vi "one.vi"() -> ()   [LabVIEW 2021]
uses:
  <vilib>/express/express analysis/Spectral/Block/exnSpectralBlock spectral measurements RMS poly.vi
  <vilib>/express/express analysis/Spectral/Block/exnSpectralBlock spectral measurements RMS DDT.vi
  <vilib>/express/express analysis/Spectral/XNode/ExpressSpectralMeasurementsBlockNode.xnode
panel:
  out "Graph in Time":dynamicdata(graph)
  out "Graph in Frequency":dynamicdata(graph)
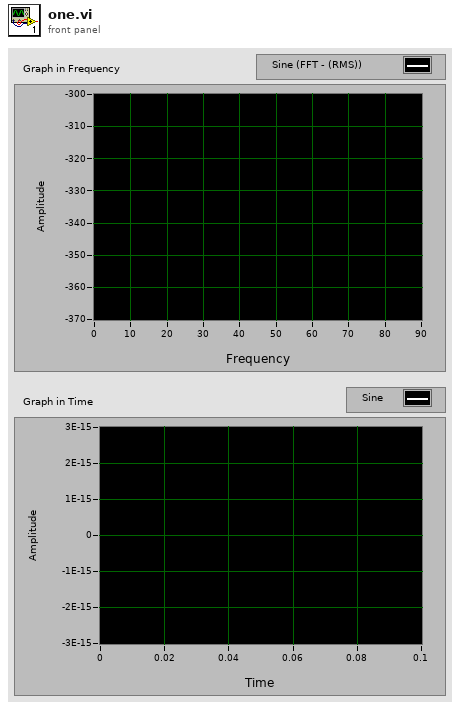
[diagram p1: front panel]
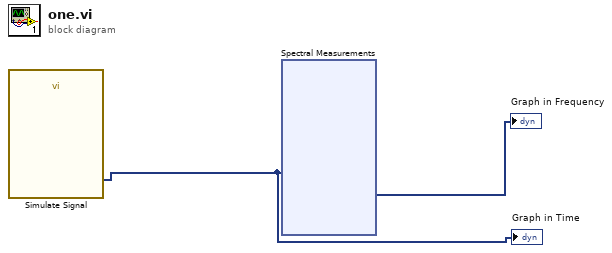
[diagram p0: block diagram]
diagram:
  n1 = call "Simulate Signal"() -> ("Sine"=w1:dynamicdata)  [unwired: 14 in, 1 out]
  "Graph in Time" <- w1
  n2 = xnode "Spectral Measurements"("Signals"=w1) -> ("FFT - (RMS)"=→"Graph in Frequency":dynamicdata)  [unwired: 1 in, 2 out]
